vi "Calc Max During Mem Fill 1.vi"(5 "StartAlgo":refnum<k21>="StartAlg2", 6 "MeanFIFO":refnum<k21>="MeanVals1", 7 "Value":fxp<+/-,22,22>, 8 "LastIterration":bool, 9 "ActiveLedIndex":u32, 10 "FirstIterration":bool, 11 "Address":u32) -> ()   [LabVIEW 2015]
uses:
  LIDAR V2 Globals.vi
  <vilib>/rvi/DataTransferAndStorage/Container/Common/niFpgaContainerExecOnDevCompGetState.vi
  <vilib>/rvi/Emulation/niFpgaEmulationIsFPGAContextNoSignature.vi
  <vilib>/rvi/Emulation/niFpgaSctlEmulationGetInTimedLoop.vi
  <vilib>/rvi/errors/niFpgaSetErrorForExecOnDevCompSimple.vi
  <vilib>/rvi/eio/common/nirviEmuReportErrorAndStop.vi
  <vilib>/rvi/DataTransferAndStorage/Container/Common/niFpgaContainerGetUniqueNameForEmu.vi
  <vilib>/rvi/FIFO/Fifo_Resource/nirvififoEmulationSetSize.vi
  <vilib>/rvi/FIFO/Fifo_Resource/nirviFifoEmulationQueueMgr.vi
  <instcachedir>/0/nirviFifoEmulationQueueMgr_E5CAEC123FF24DC58D834DCA3CDAA9B5.lvgen/nirviFifoEmulationQueueMgr_E5CAEC123FF24DC58D834DCA3CDAA9B5_001.vi
  <vilib>/rvi/FIFO/Fifo_Resource/nirvififoEmulationDetermineInputValidOut.vi
  <vilib>/rvi/FIFO/Fifo_Resource/nirvififoEmulationCreateLock.vi
  <vilib>/rvi/Emulation/niFpgaProcessEmulError.vi
  <vilib>/rvi/FIFO/Fifo_Resource/nirvififoEmulationObtainLock.vi
  <vilib>/rvi/FIFO/Fifo_Resource/nirvififoEmulationReleaseLock.vi
  <vilib>/rvi/occurrence/nirviWaitOnOccurrenceBase.vi
  <vilib>/rvi/errors/nirviReportUnexpectedCaseInternalError.vi
  <vilib>/rvi/errors/nirviReportUnexpectedCaseInternalError (U32).vi
  <vilib>/Utility/error.llb/Clear Errors.vi
  <vilib>/rvi/interface/RandomDataEmulation/niFpgaRandomDataHandleErrors.vi
  <vilib>/rvi/DataTransferAndStorage/Container/XNode/niFpgaContainer.xnode
  <vilib>/rvi/FIFO/Fifo_Resource/niFpgaFifoEmulationRefIn.vi
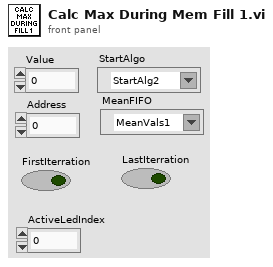
[diagram p1: front panel]
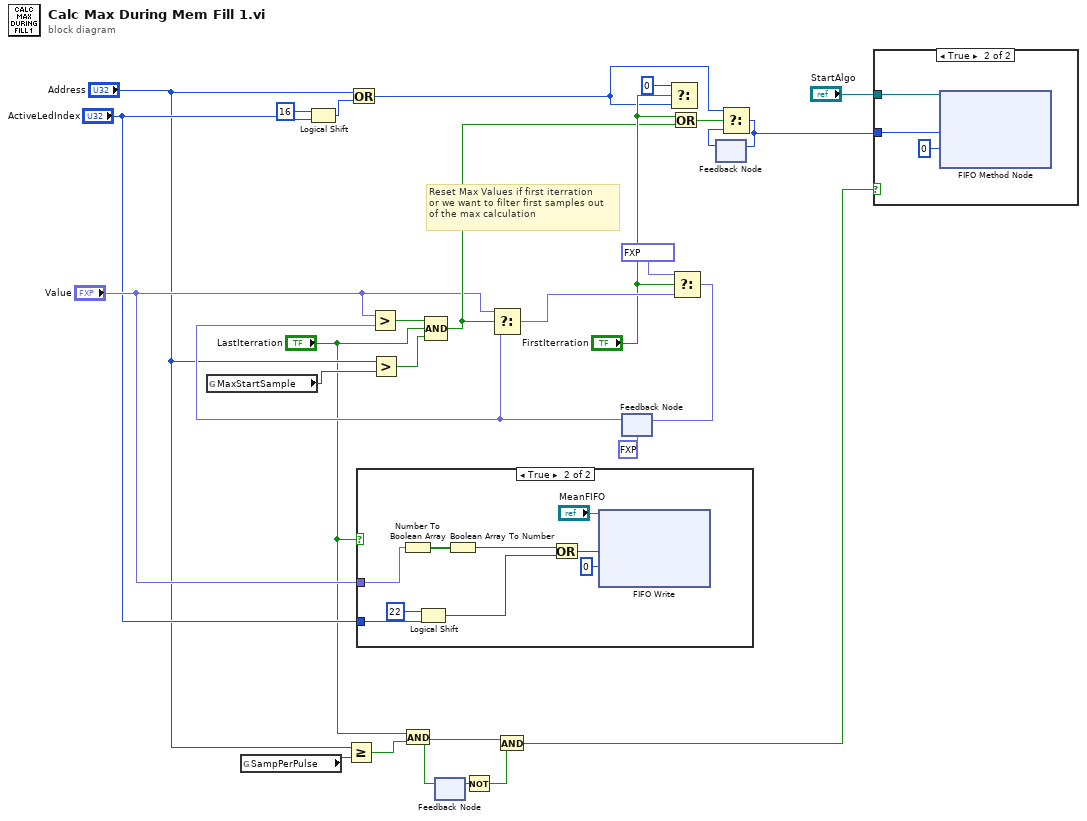
[diagram p0: block diagram]
diagram:
  # "Reset Max Values if first iterration\nor we want to filter first samples out\nof the max calculation"
  n1 = global read "LIDAR V2 Globals.vi" "MaxStartSample"() -> (w22:u32)
  n2 = global read "LIDAR V2 Globals.vi" "SampPerPulse"() -> (w10:u32)
  n3 = Logical Shift(y=i16 16, x="ActiveLedIndex") -> (x << y=w25:u32)
  n4 = Greater Or Equal?(x="Address", y=w10) -> (x >= y?=w12:bool)
  n5 = Or(x="Address", y=w25) -> (x .or. y?=w1:u32)
  n6 = case shown="True" "LastIterration" {
    tunnel: "Value" -> [_ w34]
    tunnel: "ActiveLedIndex" -> [_ w36]
    frame False {
    }
    frame True {
      n7 = Number To Boolean Array(number=w34) -> (Boolean array=w33:bool[])
      n8 = Logical Shift(y=i16 22, x=w36) -> (x << y=w35:u32)
      n9 = Boolean Array To Number(Boolean array=w33) -> (number=w32:u32)
      n10 = Or(x=w32, y=w35) -> (x .or. y?=w31:u32)
      n11 = xnode ("FIFO Write")("Element"=w31, "Timeout"=0, "FIFO In"="MeanFIFO") -> ()  [unwired: 2 out]
    }
  }
  n12 = Greater?(x="Address", y=w22) -> (0:w20:bool)
  n13 = And(x="LastIterration", y=w12) -> (x .and. y?=w8:bool)
  n14 = feedback-in #1(w8) -> ()
  n15 = feedback #1() -> (w7:bool)  [unwired: 1 in]
  n16 = Not(x=w7) -> (.not. x?=w6:bool)
  n17 = And(x=w8, y=w6) -> (x .and. y?=w5:bool)
  n18 = feedback #2(fxp<+/-,22,22> 0.0 ("Value")) -> (w18:fxp<+/-,22,22>)
  n19 = Greater?(x="Value", y=w18) -> (0:w21:bool)
  n20 = Compound Arithmetic op=AND(w21, "LastIterration", w20) -> (w15:bool)
  n21 = Select(t="Value", s=w15, f=w18) -> (s? t:f=w19:fxp<+/-,22,22>)
  n22 = Select(t=u32 0, s="FirstIterration", f=w1) -> ()  [unwired: 1 out]
  n23 = Or(x="FirstIterration", y=w15) -> (x .or. y?=w17:bool)
  n24 = Select(t=fxp<+/-,22,22> -2097152.0, s="FirstIterration", f=w19) -> (s? t:f=w28:fxp<+/-,22,22>)
  n25 = feedback-in #2(w28) -> ()
  n26 = feedback #3() -> (w4:u32)  [unwired: 1 in]
  n27 = Select(t=w1, s=w17, f=w4) -> (s? t:f=w2:u32)
  n28 = feedback-in #3(w2) -> ()
  n29 = case shown="True" w5 {
    tunnel: "StartAlgo" -> [_ w39]
    tunnel: w2 -> [_ w38]
    frame False {
    }
    frame True {
      n30 = xnode ("FIFO Method Node")("Element"=w38, "Timeout"=0, "FIFO In"=w39) -> ()  [unwired: 2 out]
    }
  }
